vi "Controller without voltage.vi"() -> ()   [LabVIEW 2014]
uses:
  Typedefs/Instructions.ctl
  Typedefs/State Information.ctl
  <vilib>/Utility/error.llb/DialogType.ctl
  Typedefs/Temperature Profile.ctl
  Typedefs/Status.ctl
  <vilib>/event_ctls.llb/usereventprio.ctl
panel:
  in  "Tab Control":enum32{"Settings", "Charts"}(tab)
  in  "Linkam Controller":refnum<visa-resource-name>="COM1"
  out "Slide":i32(slide) scale=15.0..1.0
  out "Temperature":dbl(graph)
  in  "Temperature Profile":dbl[][](array[numeric])
  out "Status":string
  out "Error":string
  out "Pump":u8
  out "°C":dbl
  in  "Start":bool
  in  "Hold":bool
  in  "Stop":bool
  in  "Disconnect":bool
  out "Current Ramp":i32
  out "Time (ms)":i32
  # "Rate(°C/min)"
  # "Hold (s)"
  # "Limit (°C)"
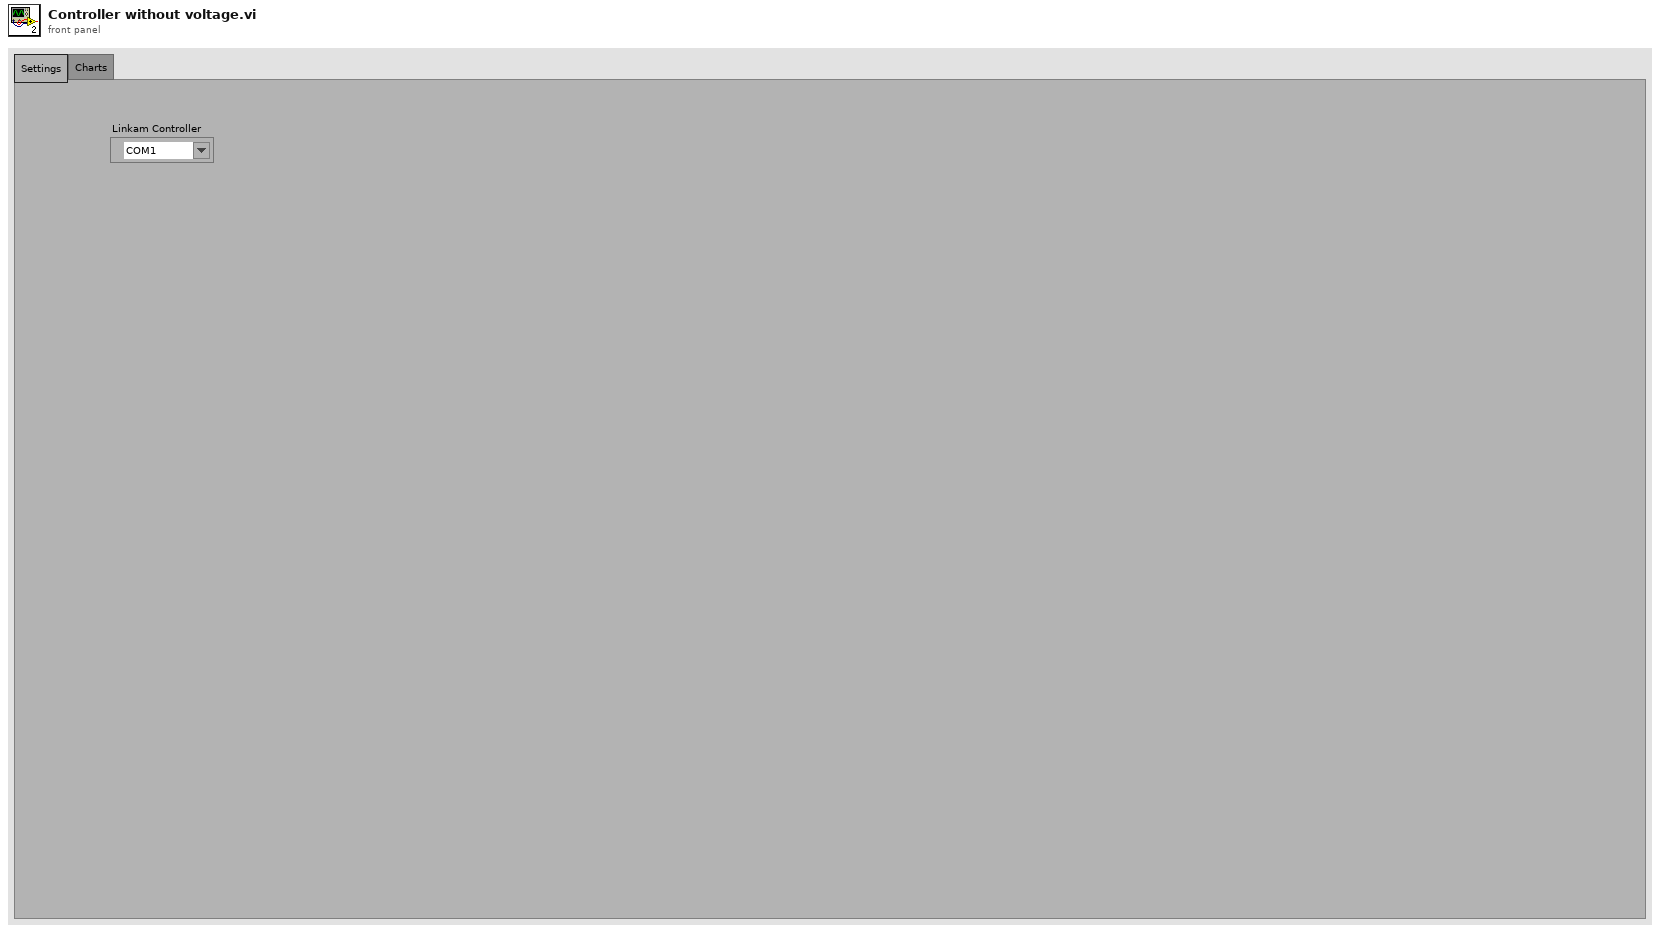
[diagram p1: front panel]
types:
  T1 = typedef "DialogType.ctl" = u16
  T2 = typedef "State Information.ctl" = cluster{"Ramp":i32, "Total Ramp":i32, "Time":i32, "Total Time":i32, "Start Time":dbl}
  T3 = typedef "Instructions.ctl" = enum16{"Idle", "Start", "Get Profile", "Go to Limit", "Hold Limit Time", "Stop", "Disconnect"}
  T4 = typedef "Temperature Profile.ctl" = enum16{"Rate", "Limit", "Hold Time"}
  T5 = typedef "Status.ctl" = enum16{"No Status", "Stopped", "Heating", "Cooling", "Limit Reached", "Holding the Limit Time", "Manual Hold"}
  T6 = typedef "usereventprio.ctl" = enum32{"high priority", "normal priority"}
  T7 = cluster{"Temperature":dbl, "Status":string, "Error":string, "Pump":u8}
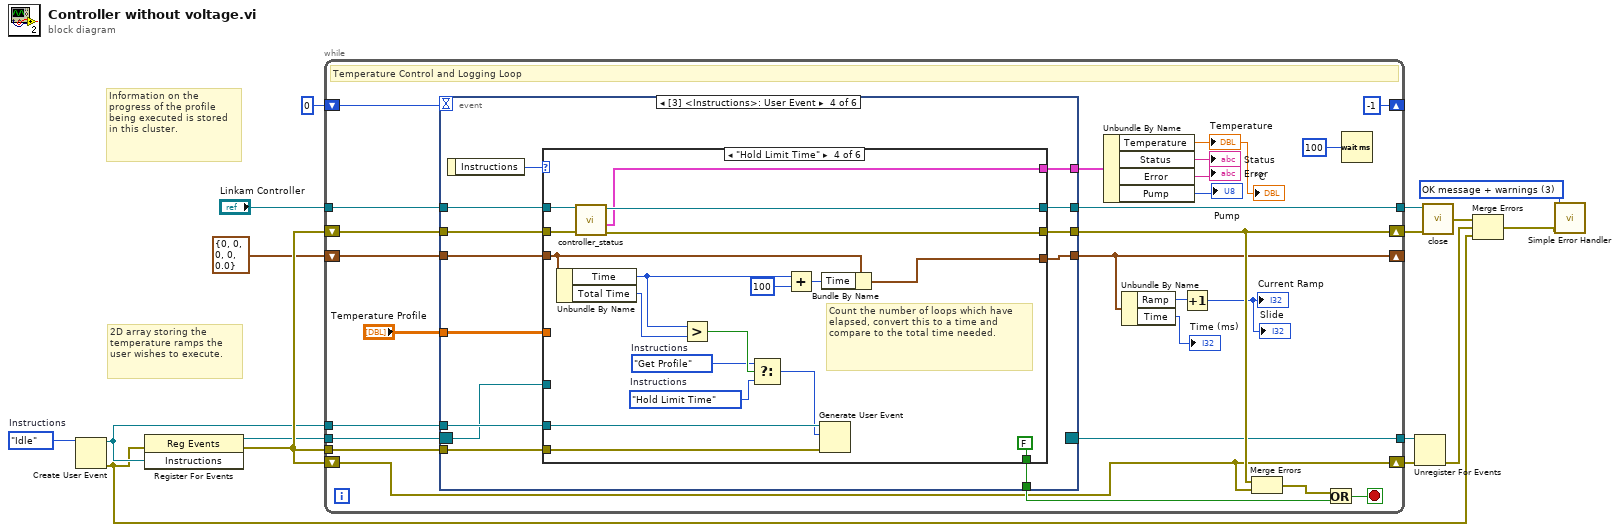
[diagram p0: block diagram]
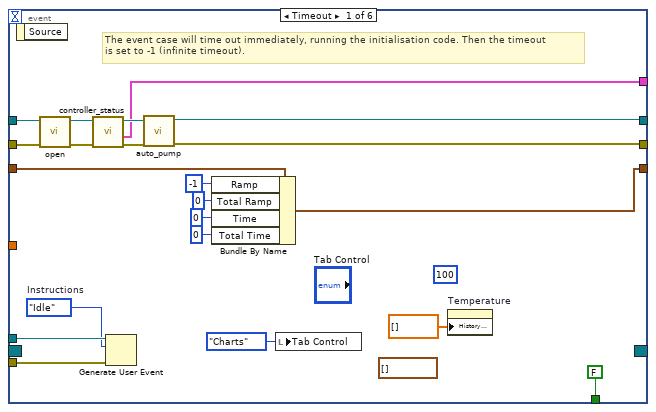
[diagram p2: hidden frame]
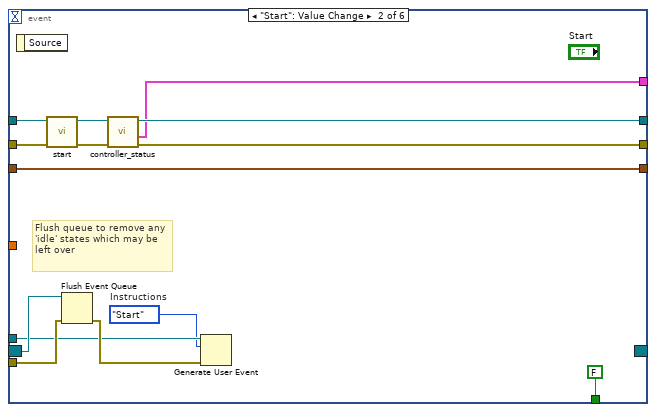
[diagram p3: hidden frame]
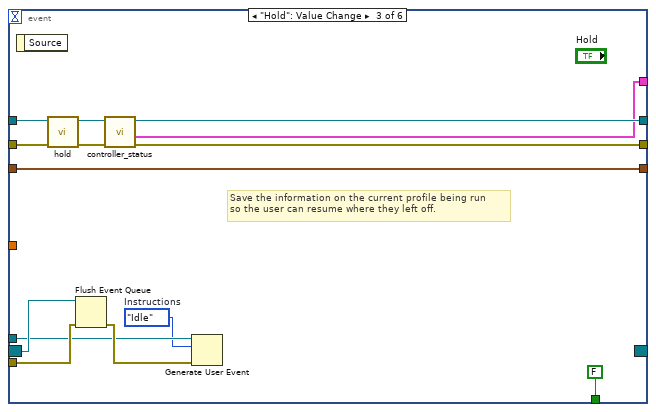
[diagram p4: hidden frame]
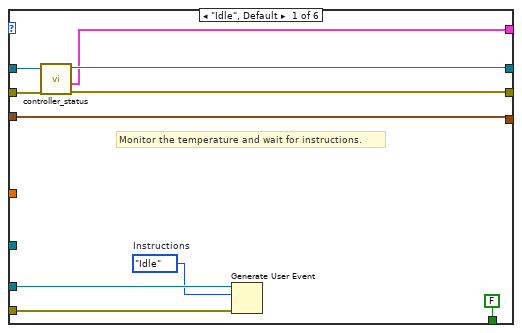
[diagram p5: hidden frame]
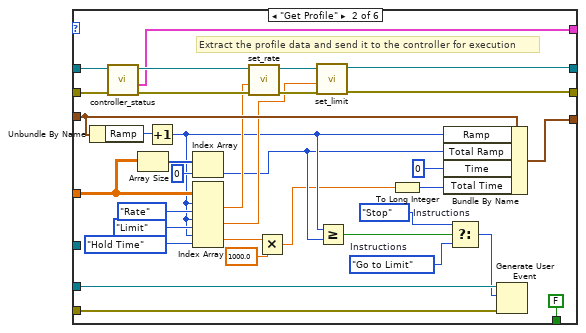
[diagram p6: hidden frame]
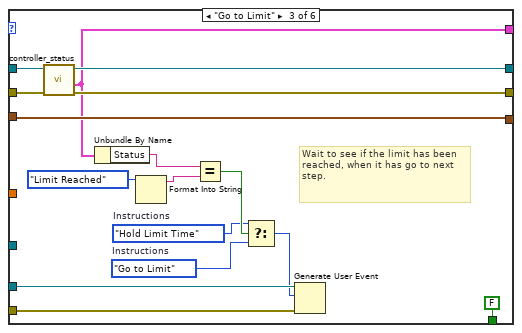
[diagram p7: hidden frame]
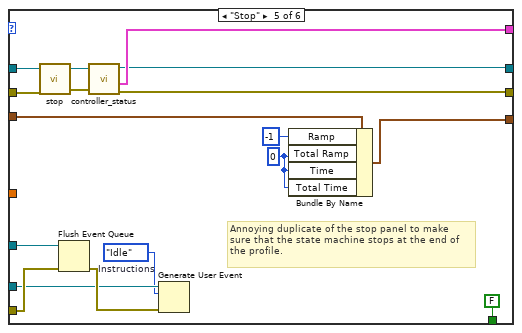
[diagram p8: hidden frame]
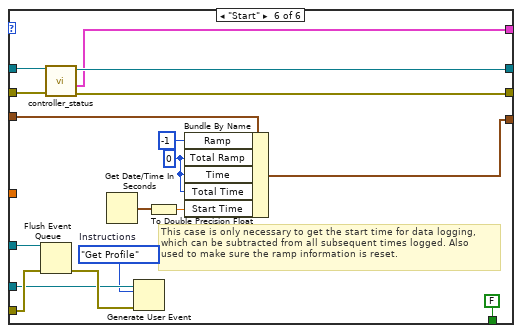
[diagram p9: hidden frame]
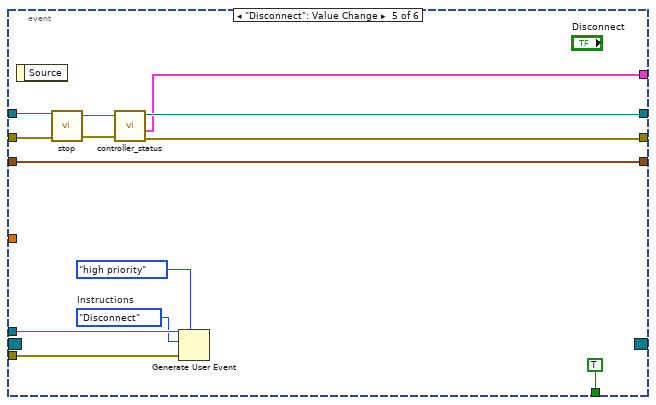
[diagram p10: hidden frame]
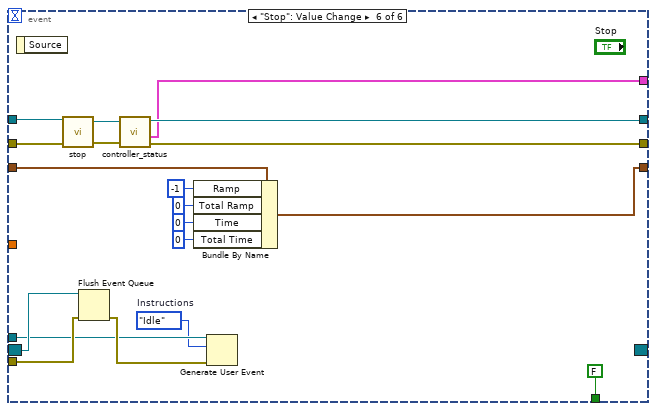
[diagram p11: hidden frame]
diagram:
  w2 = T1 3 items=["no dialog", "OK message", "continue or stop message", "OK message + warnings", "continue/stop + warnings"] ("type of dialog (OK msg:1)")
  w14 = Instructions."Idle"  # Instructions
  # "Information on the progress of the profile being executed is stored in this cluster."
  # "2D array storing the temperature ramps the user wishes to execute."
  n1 = Create User Event(user event datatype=w14) -> (user event=w6:refnum<user-event>, error out=w3:errorcluster)  [unwired: 1 in]
  n2 = register-events(error in=w3, w6) -> (reference out=w15:refnum<event-registration>, error out=w16:errorcluster)  [unwired: 1 in]
  n3 = while {
    tunnel: w15 -> [w41]
    tunnel: [w40] -> w13
    shift-right: [w25] -> w12
    shift-left: w16 -> [w25]
    tunnel: "Linkam Controller" -> [w37]
    tunnel: [w35] -> w10
    shift-right: [w42] -> w9
    shift-left: w16 -> [w36]
    tunnel: w6 -> [w34]
    shift-right: [w23] -> _
    shift-left: T2 {"Ramp"=0, "Total Ramp"=0, "Time"=0, "Total Time"=0, "Start Time"=0.0} ("State Information") -> [w33]
    tunnel: w16 -> [w32]
    shift-right: [-1] -> _
    shift-left: 0 -> [w20]
    stop <- w39 stop-if-true
    # "Temperature Control and Logging Loop"
    n4 = event shown="[3] <Instructions>: User Event" {
      selector: w41 -> [_ w68 w90 w92 _ w240]
      dyn-events: [_ _ _ _ _ _] -> w40
      timeout: w20 -> [_ _ _ _ _ _]
      tunnel: [FALSE FALSE FALSE w103 TRUE FALSE] -> w38
      tunnel: w37 -> [w60 w76 w85 w102 w228 w237]
      tunnel: w36 -> [w59 w77 w84 w101 w229 w236]
      tunnel: [w53 w73 w81 w100 w225 w233] -> w35
      tunnel: [w52 w72 w80 w99 w224 w232] -> w42
      tunnel: w34 -> [w63 w67 w87 w98 w221 w239]
      tunnel: w33 -> [w47 w64 w78 w97 w222 w246]
      tunnel: [w46 w64 w78 w96 w222 w245] -> w23
      tunnel: w32 -> [w62 w70 w89 w95 w220 w247]
      tunnel: "Temperature Profile" -> [_ _ _ w94 _ _]
      tunnel: [w54 w71 w79 w93 w223 w231] -> w17
      event Timeout {
        (unwired) waveform(dbl)[] [] ("History Data")
        (unwired) u32 100 ("Temp loop delay")
        w61 = Instructions."Idle"  # Instructions
        # "The event case will time out immediately, running the initialisation code. Then the timeout\nis set to -1 (infinite timeout)."
        n5 = event-data() -> ()  [unwired: 1 in, 1 out]
        n6 = call "open.vi"("error in (no error)"=w59, "reference"=w60) -> ("error out"=w58:errorcluster, "reference out"=w57:refnum<visa-resource-name>)  [unwired: 8 in]
        n7 = call "controller_status.vi"("error in (no error)"=w58, "VISA Refnum in"=w57) -> ("error out"=w56:errorcluster, "output cluster"=w54:T7, "VISA Refnum out"=w55:refnum<visa-resource-name>)  [unwired: 7 in]
        n8 = Generate User Event(user event=w63, event data cluster=w61, error in=w62) -> ()  [unwired: 1 in, 2 out]
        n9 = call "auto_pump.vi"("error in (no error)"=w56, "VISA Refnum in"=w55) -> ("error out"=w52:errorcluster, "VISA Refnum out"=w53:refnum<visa-resource-name>)  [unwired: 8 in]
        n10 = Bundle By Name(cluster=w47, "Ramp"=-1, "Total Ramp"=0, "Time"=0, "Total Time"=0) -> (w46:T2)
        n11 = local write "Tab Control"(enum32{"Settings", "Charts"}."Charts" ("Tab Control")) -> ()
        n12 = property on="Temperature" class="WFChart (strict)"("History Data"=dbl[] []) -> ()  [unwired: 2 in, 2 out]
      }
      event "Start": Value Change {
        w66 = Instructions."Start"  # Instructions
        # "Flush queue to remove any 'idle' states which may be left over"
        n13 = event-data() -> ()  [unwired: 1 in, 1 out]
        n14 = call "start.vi"("error in (no error)"=w77, "VISA resource name"=w76) -> ("Error out"=w74:errorcluster, "VISA resource name out"=w75:refnum<visa-resource-name>)  [unwired: 4 in]
        n15 = Flush Event Queue(0:w68, 3:w70) -> (11:w69:errorcluster)  [unwired: 4 in, 2 out]
        n16 = call "controller_status.vi"("error in (no error)"=w74, "VISA Refnum in"=w75) -> ("error out"=w72:errorcluster, "output cluster"=w71:T7, "VISA Refnum out"=w73:refnum<visa-resource-name>)  [unwired: 7 in]
        n17 = Generate User Event(user event=w67, event data cluster=w66, error in=w69) -> ()  [unwired: 1 in, 2 out]
      }
      event "Hold": Value Change {
        w86 = Instructions."Idle"  # Instructions
        # "Save the information on the current profile being run\nso the user can resume where they left off."
        n18 = event-data() -> ()  [unwired: 1 in, 1 out]
        n19 = call "hold.vi"("error in (no error)"=w84, "VISA resource name"=w85) -> ("error out"=w82:errorcluster, "VISA resource name out"=w83:refnum<visa-resource-name>)  [unwired: 4 in]
        n20 = Flush Event Queue(0:w90, 3:w89) -> (11:w88:errorcluster)  [unwired: 4 in, 2 out]
        n21 = call "controller_status.vi"("error in (no error)"=w82, "VISA Refnum in"=w83) -> ("error out"=w80:errorcluster, "output cluster"=w79:T7, "VISA Refnum out"=w81:refnum<visa-resource-name>)  [unwired: 7 in]
        n22 = Generate User Event(user event=w87, event data cluster=w86, error in=w88) -> ()  [unwired: 1 in, 2 out]
      }
      event User Event {
        n23 = event-data() -> ("Instructions"=w104:T3)  [unwired: 1 in]
        n24 = case shown="\"Hold Limit Time\"" w104 {
          tunnel: [FALSE FALSE FALSE FALSE FALSE FALSE] -> w103
          tunnel: w102 -> [w113 w147 w163 w181 w199 w209]
          tunnel: w101 -> [w114 w148 w164 w182 w198 w210]
          tunnel: [w112 w142 w162 w180 w194 w208] -> w100
          tunnel: [w111 w141 w161 w179 w193 w207] -> w99
          tunnel: w98 -> [w108 w121 w159 w176 w188 w201]
          tunnel: w97 -> [w109 w132 w150 w171 w192 w216]
          tunnel: [w109 w130 w150 w170 w191 w211] -> w96
          tunnel: w95 -> [w107 w120 w158 w175 w190 w203]
          tunnel: w94 -> [_ w135 _ _ _ _]
          tunnel: [w105 w118 w149 w166 w195 w206] -> w93
          tunnel: w92 -> [_ _ _ _ w187 w204]
          frame "Idle", Default {
            w106 = Instructions."Idle"  # Instructions
            # "Monitor the temperature and wait for instructions."
            n25 = call "controller_status.vi"("error in (no error)"=w114, "VISA Refnum in"=w113) -> ("error out"=w111:errorcluster, "output cluster"=w105:T7, "VISA Refnum out"=w112:refnum<visa-resource-name>)  [unwired: 7 in]
            n26 = Generate User Event(user event=w108, event data cluster=w106, error in=w107) -> ()  [unwired: 1 in, 2 out]
          }
          frame "Get Profile" {
            w123 = Instructions."Stop"  # Instructions
            w122 = Instructions."Go to Limit"  # Instructions
            # "Extract the profile data and send it to the controller for execution"
            n27 = Unbundle By Name(w132) -> ("Ramp"=w139:i32)
            n28 = call "controller_status.vi"("error in (no error)"=w148, "VISA Refnum in"=w147) -> ("error out"=w145:errorcluster, "output cluster"=w118:T7, "VISA Refnum out"=w146:refnum<visa-resource-name>)  [unwired: 7 in]
            n29 = Array Size(array=w135) -> (size(s)=w134:i32[])
            n30 = Increment(x=w139) -> (x+1=w126:i32)
            n31 = Index Array(array=w134, index=0) -> (element=w125:i32)
            n32 = Index Array(array=w135, index (row) #1=w126, index (col) #1=Temperature_Profile."Rate" ("Enum"), index (row) #2=w126, index (col) #2=Temperature_Profile."Limit" ("Enum"), index (row) #3=w126, index (col) #3=Temperature_Profile."Hold Time" ("Enum")) -> (element #1=w128:dbl, element #2=w127:dbl, element #3=w117:dbl)
            n33 = call "set_rate.vi"("error in (no error)"=w145, "Set Rate"=w128, "VISA resource name in"=w146) -> ("error out"=w143:errorcluster, "VISA resource name out"=w144:refnum<visa-resource-name>)  [unwired: 3 in]
            n34 = Multiply(x=w117, y=1000.0) -> (x*y=w115:dbl)
            n35 = call "set_limit.vi"("error in (no error)"=w143, "Set Temperature"=w127, "VISA resource name"=w144) -> ("error out"=w141:errorcluster, "VISA resource name out"=w142:refnum<visa-resource-name>)  [unwired: 3 in]
            n36 = Greater Or Equal?(x=w126, y=w125) -> (x >= y?=w124:bool)
            n37 = To Long Integer(number=w115) -> (32bit integer=w116:i32)
            n38 = Bundle By Name(cluster=w132, "Ramp"=w126, "Total Ramp"=w125, "Time"=0, "Total Time"=w116) -> (w130:T2)
            n39 = Select(t=w123, s=w124, f=w122) -> (s? t:f=w119:T3)
            n40 = Generate User Event(user event=w121, event data cluster=w119, error in=w120) -> ()  [unwired: 1 in, 2 out]
          }
          frame "Go to Limit" {
            w152 = Instructions."Go to Limit"  # Instructions
            w153 = Instructions."Hold Limit Time"  # Instructions
            # "Wait to see if the limit has been reached, when it has go to next step."
            n41 = call "controller_status.vi"("error in (no error)"=w164, "VISA Refnum in"=w163) -> ("error out"=w161:errorcluster, "output cluster"=w149:T7, "VISA Refnum out"=w162:refnum<visa-resource-name>)  [unwired: 7 in]
            n42 = Unbundle By Name(w149) -> ("Status"=w156:string)
            n43 = Format Into String(Status."Limit Reached" ("Enum")) -> (resulting string=w155:string)  [unwired: 3 in, 1 out]
            n44 = Equal?(x=w156, y=w155) -> (x = y?=w154:bool)
            n45 = Select(t=w153, s=w154, f=w152) -> (s? t:f=w151:T3)
            n46 = Generate User Event(user event=w159, event data cluster=w151, error in=w158) -> ()  [unwired: 1 in, 2 out]
          }
          frame "Hold Limit Time" {
            w172 = Instructions."Hold Limit Time"  # Instructions
            w173 = Instructions."Get Profile"  # Instructions
            # "Count the number of loops which have elapsed, convert this to a time and compare to the total time needed."
            n47 = Unbundle By Name(w171) -> ("Time"=w169:i32, "Total Time"=w177:i32)
            n48 = call "controller_status.vi"("error in (no error)"=w182, "VISA Refnum in"=w181) -> ("error out"=w179:errorcluster, "output cluster"=w166:T7, "VISA Refnum out"=w180:refnum<visa-resource-name>)  [unwired: 7 in]
            n49 = Greater?(x=w169, y=w177) -> (0:w174:bool)
            n50 = Select(t=w173, s=w174, f=w172) -> (s? t:f=w168:T3)
            n51 = Add(x=w169, y=100) -> (x+y=w167:i32)
            n52 = Generate User Event(user event=w176, event data cluster=w168, error in=w175) -> ()  [unwired: 1 in, 2 out]
            n53 = Bundle By Name(cluster=w171, "Time"=w167) -> (w170:T2)
          }
          frame "Stop" {
            w183 = 0 ("Total Ramp")
            w186 = Instructions."Idle"  # Instructions
            # "Annoying duplicate of the stop panel to make\nsure that the state machine stops at the end of\nthe profile."
            n54 = call "stop.vi"("VISA resource name"=w199, "error in (no error)"=w198) -> ("VISA resource name out"=w196:refnum<visa-resource-name>, "Error out"=w197:errorcluster)  [unwired: 6 in]
            n55 = Flush Event Queue(0:w187, 3:w190) -> (11:w189:errorcluster)  [unwired: 4 in, 2 out]
            n56 = call "controller_status.vi"("error in (no error)"=w197, "VISA Refnum in"=w196) -> ("error out"=w193:errorcluster, "output cluster"=w195:T7, "VISA Refnum out"=w194:refnum<visa-resource-name>)  [unwired: 7 in]
            n57 = Generate User Event(user event=w188, event data cluster=w186, error in=w189) -> ()  [unwired: 1 in, 2 out]
            n58 = Bundle By Name(cluster=w192, "Ramp"=-1, "Total Ramp"=w183, "Time"=w183, "Total Time"=w183) -> (w191:T2)
          }
          frame "Start" {
            w200 = Instructions."Get Profile"  # Instructions
            w212 = 0 ("Total Ramp")
            # "This case is only necessary to get the start time for data logging,\nwhich can be subtracted from all subsequent times logged. Also\nused to make sure the ramp information is reset."
            n59 = Flush Event Queue(0:w204, 3:w203) -> (11:w202:errorcluster)  [unwired: 4 in, 2 out]
            n60 = call "controller_status.vi"("error in (no error)"=w210, "VISA Refnum in"=w209) -> ("error out"=w207:errorcluster, "output cluster"=w206:T7, "VISA Refnum out"=w208:refnum<visa-resource-name>)  [unwired: 7 in]
            n61 = Get Date/Time In Seconds() -> (seconds since 1Jan1904=w214:timestamp)
            n62 = Generate User Event(user event=w201, event data cluster=w200, error in=w202) -> ()  [unwired: 1 in, 2 out]
            n63 = To Double Precision Float(number=w214) -> (double precision float=w215:dbl)
            n64 = Bundle By Name(cluster=w216, "Ramp"=-1, "Total Ramp"=w212, "Time"=w212, "Total Time"=w212, "Start Time"=w215) -> (w211:T2)
          }
        }
      }
      event "Disconnect": Value Change {
        w218 = Instructions."Disconnect"  # Instructions
        n65 = event-data() -> ()  [unwired: 1 in, 1 out]
        n66 = call "stop.vi"("VISA resource name"=w228, "error in (no error)"=w229) -> ("VISA resource name out"=w227:refnum<visa-resource-name>, "Error out"=w226:errorcluster)  [unwired: 6 in]
        n67 = call "controller_status.vi"("error in (no error)"=w226, "VISA Refnum in"=w227) -> ("error out"=w224:errorcluster, "output cluster"=w223:T7, "VISA Refnum out"=w225:refnum<visa-resource-name>)  [unwired: 7 in]
        n68 = Generate User Event(priority (normal)=usereventprio."high priority", user event=w221, event data cluster=w218, error in=w220) -> ()  [unwired: 2 out]
      }
      event "Stop": Value Change {
        w238 = Instructions."Idle"  # Instructions
        n69 = event-data() -> ()  [unwired: 1 in, 1 out]
        n70 = call "stop.vi"("VISA resource name"=w237, "error in (no error)"=w236) -> ("VISA resource name out"=w234:refnum<visa-resource-name>, "Error out"=w235:errorcluster)  [unwired: 6 in]
        n71 = Flush Event Queue(0:w240, 3:w247) -> (11:w248:errorcluster)  [unwired: 4 in, 2 out]
        n72 = call "controller_status.vi"("error in (no error)"=w235, "VISA Refnum in"=w234) -> ("error out"=w232:errorcluster, "output cluster"=w231:T7, "VISA Refnum out"=w233:refnum<visa-resource-name>)  [unwired: 7 in]
        n73 = Bundle By Name(cluster=w246, "Ramp"=-1, "Total Ramp"=0, "Time"=0, "Total Time"=0) -> (w245:T2)
        n74 = Generate User Event(user event=w239, event data cluster=w238, error in=w248) -> ()  [unwired: 1 in, 2 out]
      }
    }
    n75 = Unbundle By Name(w17) -> ("Temperature"=→"Temperature" →"°C":dbl, "Status"=→"Status":string, "Error"=→"Error":string, "Pump"=→"Pump":u8)
    n76 = Unbundle By Name(w23) -> ("Ramp"=w21:i32, "Time"=→"Time (ms)":i32)
    n77 = Increment(x=w21) -> (x+1=→"Current Ramp" →"Slide":i32)
    n78 = Merge Errors(w42, w25) -> (w24:errorcluster)
    n79 = Or(x=w24, y=w38) -> (x .or. y?=w39:bool)
    n80 = Wait (ms)(milliseconds to wait=u32 100 ("Temp loop delay")) -> ()  [unwired: 1 out]
  }
  n81 = Unregister For Events(event registration refnum=w13, error in=w12) -> (error out=w4:errorcluster)
  n82 = call "close.vi"("Error in"=w9, "VISA resource name"=w10) -> ("Error out"=w5:errorcluster)  [unwired: 2 in]
  n83 = Merge Errors(w5, w4, w3) -> (w1:errorcluster)
  n84 = call <vilib>:"Simple Error Handler.vi"("type of dialog (OK msg:1)"=w2, "error in (no error)"=w1) -> ()  [unwired: 3 in, 5 out]
